vi "Read Created Attributes.vi"(10 "Alias":string, 11 "TEMPLATE Actor in":refnum<class "TEMPLATE Actor.lvclass">) -> (0 "Error out":errorcluster, 2 "Created Attributes":refnum<class "Attributes.lvclass">)   [LabVIEW 2025, in "TEMPLATE Actor.lvlib" / "TEMPLATE Actor.lvclass"]
uses:
  TEMPLATE Actor.lvclass
  <vilib>/Nathan Davis/jettl/jettl/jettl/Attributes/Attributes/Attributes.lvclass
  TEMPLATE Actor.lvclass/TEMPLATE Actor.ctl
  <vilib>/Nathan Davis/jettl/jettl/jettl/Actor/Actor/Actor.lvclass
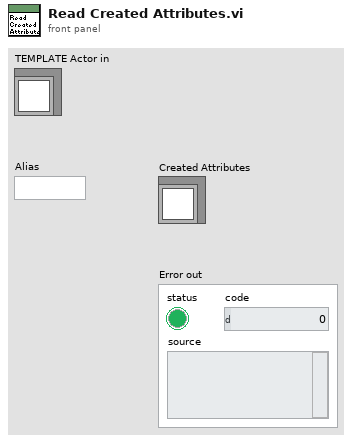
[diagram p1: front panel]
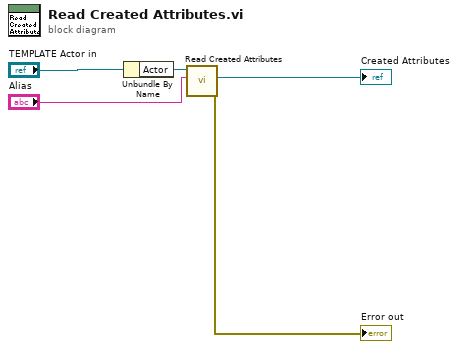
[diagram p0: block diagram]
diagram:
  n1 = Unbundle By Name("TEMPLATE Actor in") -> ("Actor"=w5:refnum<class "Actor.lvclass">)
  n2 = call-dynamic "Read Created Attributes.vi"("Alias"="Alias", "Actor in"=w5) -> ("Error out"=→"Error out":errorcluster, "Created Attributes"=→"Created Attributes":refnum<class "Attributes.lvclass">)  [unwired: 8 in]
